vi "Instruction List Start Address.vi"(6 "Starting Address Offset":u16 format="%04x", 7 "Virtual Memory Unit in":refnum<class "Virtual Memory Unit.lvclass">, 8 "error in (no error)":errorcluster, 11 "Bus Controller in":refnum<class "Bus Controller.lvclass">) -> (0 "error out":errorcluster, 3 "Bus Controller out":refnum<class "Bus Controller.lvclass">, 5 "Virtual Memory Unit out":refnum<class "Virtual Memory Unit.lvclass">)   [LabVIEW 2020, in "BCI-1553 API.lvlib" / "Bus Controller.lvclass"]
doc: "Sets the instruction list starting address for this Bus Controller."
uses:
  Bus Controller.lvclass
  Dependencies/Virtual Memory Unit/Virtual Memory Unit.lvclass
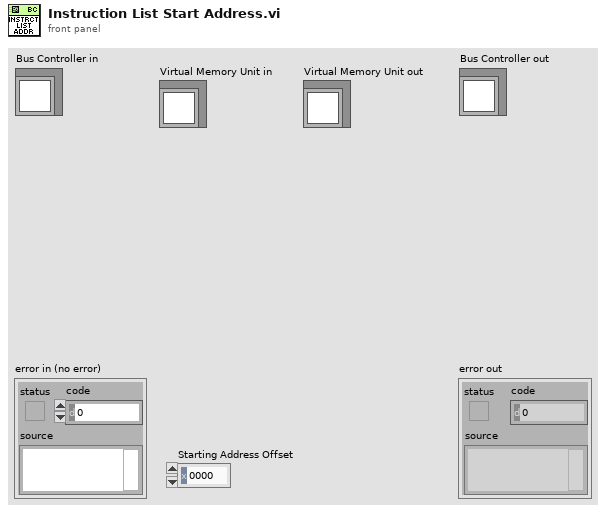
[diagram p1: front panel]
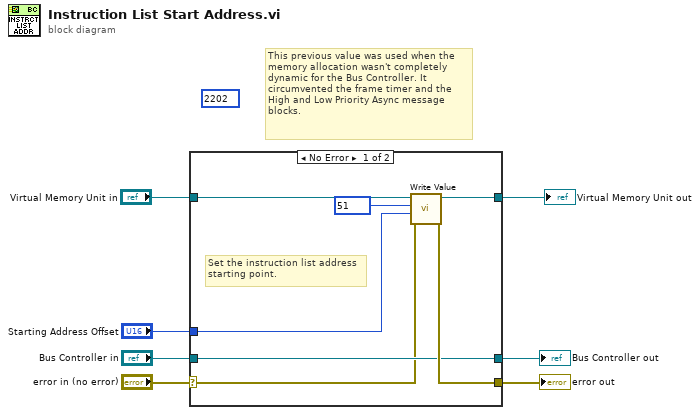
[diagram p0: block diagram]
diagram:
  (unwired) u16 2202 ("Address")
  # "This previous value was used when the\nmemory allocation wasn't completely\ndynamic for the Bus Controller. It \ncircumvented the frame timer and the\nHigh and Low Priority Async message\nblocks."
  n1 = case shown="No Error" "error in (no error)" {
    selector: "error in (no error)" -> [w10 w17]
    tunnel: [w14 w17] -> w2
    tunnel: [w13 w16] -> w5
    tunnel: "Bus Controller in" -> [w13 w16]
    tunnel: "Virtual Memory Unit in" -> [w12 w15]
    tunnel: [w11 w15] -> w4
    tunnel: "Starting Address Offset" -> [w8 _]
    frame No Error {
      # "Set the instruction list address\nstarting point."
      n2 = call "Write Value.vi"("error in (no error)"=w10, "Value"=w8, "Index"=51 ("Address"), "Virtual Memory Unit in"=w12) -> ("error out"=w14:errorcluster, "Virtual Memory Unit out"=w11:refnum<class "Virtual Memory Unit.lvclass">)  [unwired: 6 in]
    }
    frame Error {
    }
  }
  "error out" <- w2
  "Bus Controller out" <- w5
  "Virtual Memory Unit out" <- w4
